vi "G#Object_NewClassAttributes.vi"(0 "reference in":refnum<class "G#Object.lvclass">, 3 "check if valid only (F)":bool, 5 "error in (no error)":errorcluster) -> (14 "reference out":refnum<class "G#Object.lvclass">, 16 "static attribute ref":u32, 17 "created new":bool, 18 "valid":bool, 19 "error out":errorcluster)   [LabVIEW 2017, in "G#Object.lvclass"]
doc: "Creates a new object, but will also make it possible for the debugger process to create the object instead, this way, the debugger will own all of the queues and data value reference and single stepping of methods are possible."
uses:
  G#Object.lvclass
  G#Object_State.ctl
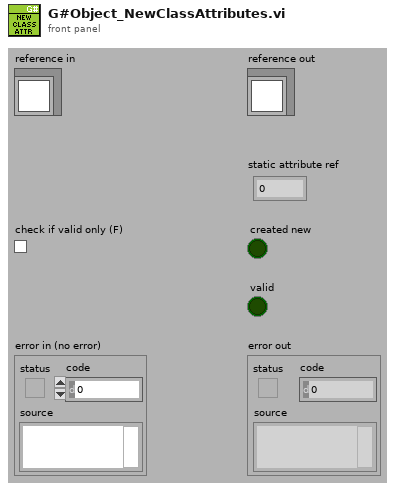
[diagram p1: front panel]
types:
  T1 = typedef "G#Object.lvclass/G#Object_State.ctl" = enum16{"Clear", "Create", "Delete", "Get class attributes", "Class hierarchy", "Get attribute value", "Set attribute value"}
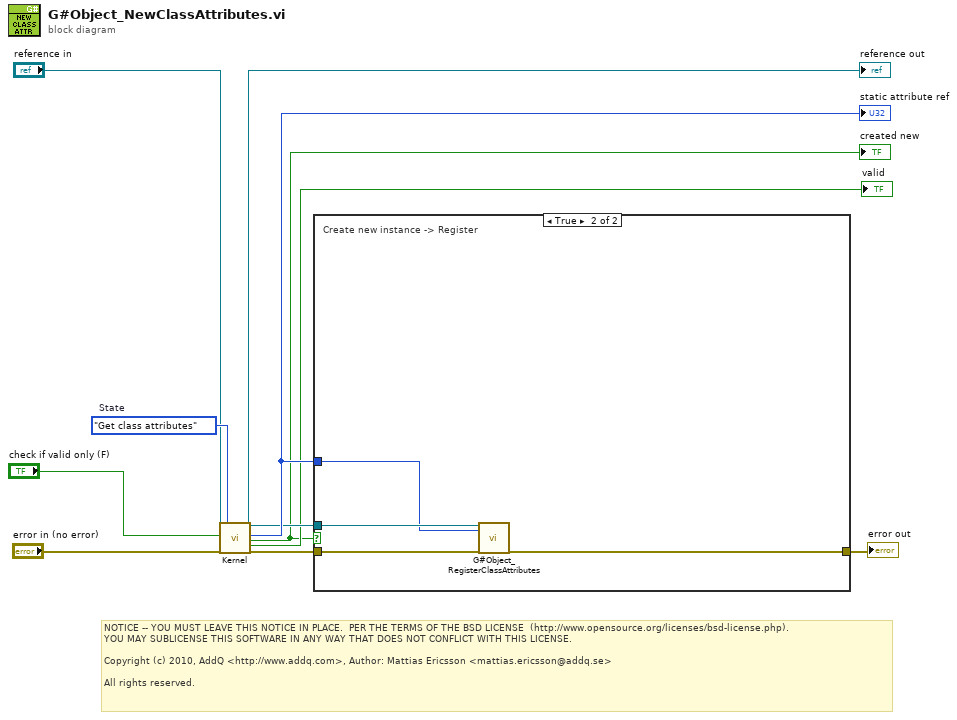
[diagram p0: block diagram]
diagram:
  w9 = G#Object_State."Get class attributes"  # State
  # "NOTICE -- YOU MUST LEAVE THIS NOTICE IN PLACE.  PER THE TERMS OF THE BSD LICENSE  (http://www.opensource.org/licenses/bsd-license.php).\nYOU MAY SUBLICENSE THIS SOFTWARE IN ANY WAY THAT DOES NOT CONFLICT WITH THIS LICENSE.\n\nCopyright (c) 2010, AddQ <http://www.addq.com>, Author: Mattias Ericsson <mattias.ericsson@addq.se>\n\nAll rights reserved."
  n1 = call-dynamic "Kernel.vi"("reference in"="reference in", "option 1"="check if valid only (F)", "error in (no error)"="error in (no error)", "state"=w9) -> ("reference out"=w4:refnum<class "G#Object.lvclass">, "static attribute ref"=w6:u32, "output 1"=w1:bool, "output 2"=→"valid":bool, "error out"=w5:errorcluster)  [unwired: 7 in, 4 out]
  "reference out" <- w4
  "static attribute ref" <- w6
  "created new" <- w1
  n2 = case shown="True" w1 {
    tunnel: [w11 w14] -> w7
    tunnel: w6 -> [_ w12]
    tunnel: w5 -> [w11 w15]
    tunnel: w4 -> [_ w13]
    frame False {
    }
    frame True {
      # "Create new instance -> Register"
      n3 = call "G#Object_RegisterClassAttributes.vi"("reference in"=w13, "static attribute ref"=w12, "error in (no error)"=w15) -> ("error out"=w14:errorcluster)  [unwired: 15 in, 1 out]
    }
  }
  "error out" <- w7
